vi "dfd_Sampled FFT.vi"(7 "# freq bins (512)":i32=512, 11 "h[n]":dbl[](array[numeric]) format="%.2f") -> (3 "FFT {X}":cdb[](array[numeric]) format="%.2f")   [LabVIEW 2017, in "NI_DigFilterLicensed.lvlib"]
uses:
  <vilib>/addons/Digital Filter Design/NI_DigFilterLicensed.lvlib
  <vilib>/Analysis/2dsp.llb/Real FFT.vi
  <vilib>/Analysis/NI_AALPro.lvlib
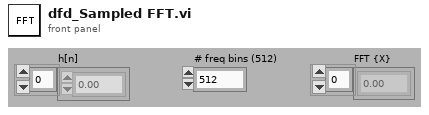
[diagram p1: front panel]
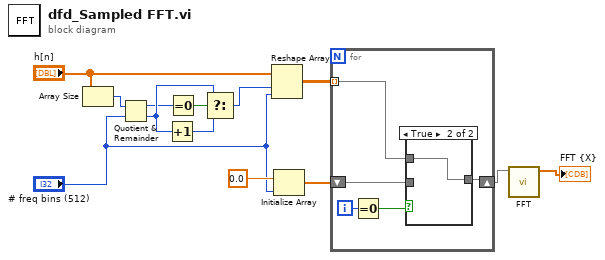
[diagram p0: block diagram]
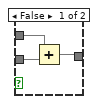
[diagram p2: hidden frame]
diagram:
  n1 = Array Size(array="h[n]") -> (size(s)=w13:i32)
  n2 = Quotient & Remainder(x=w13, y="# freq bins (512)") -> (x-y*floor(x/y)=w6:i32, floor(x/y)=w9:i32)
  n3 = Increment(x=w9) -> (x+1=w8:i32)
  n4 = Equal To 0?(x=w6) -> (x = 0?=w7:bool)
  n5 = Select(t=w9, s=w7, f=w8) -> (s? t:f=w1:i32)
  n6 = Reshape Array("h[n]", w1, "# freq bins (512)") -> (w11:dbl[][])
  n7 = Initialize Array(0.0, "# freq bins (512)") -> (w10:dbl[])
  n8 = for {
    shift-right: [w16] -> w3
    shift-left: w10 -> [w14]
    tunnel: w11 -> [w15] mode=indexing
    i -> [w18]
    n9 = Equal To 0?(x=w18) -> (x = 0?=w17:bool)
    n10 = case shown="True" w17 {
      tunnel: [w19 w22] -> w16
      tunnel: w15 -> [w20 w22]
      tunnel: w14 -> [w21 _]
      frame False {
        n11 = Add(x=w20, y=w21) -> (x+y=w19:dbl[])
      }
      frame True {
      }
    }
  }
  n12 = call-poly <vilib>:"FFT.vi"("X"=w3) -> ("FFT {X}"=→"FFT {X}":cdb[])  [unwired: 2 in, 8 out]
